vi "_sub_raw_data_analysis.vi"(11 "raw data input":u32[](array[numeric])) -> (1 "Raw-Del":u32[](array[numeric]), 2 "MAX":u32, 3 "raw data output":u32[](array[numeric]), 4 "LWA_DEL":u32, 5 "MIN":u32)   [LabVIEW 2015]
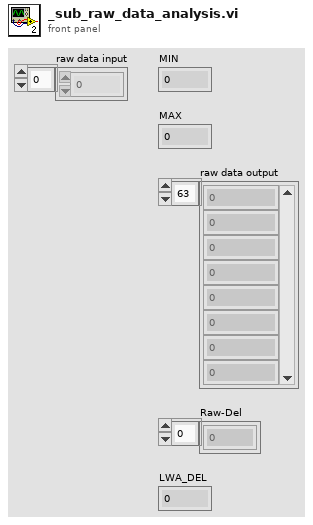
[diagram p1: front panel]
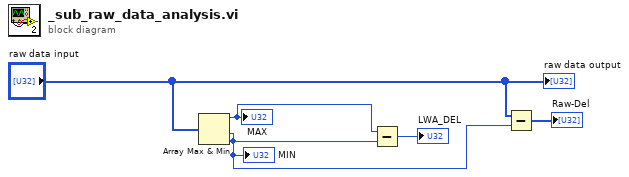
[diagram p0: block diagram]
diagram:
  n1 = Array Max & Min(array="raw data input") -> (max value=w1:u32, min value=w4:u32)  [unwired: 2 out]
  "MAX" <- w1
  "MIN" <- w4
  n2 = Subtract(x=w1, y=w4) -> (x-y=→"LWA_DEL":u32)
  n3 = Subtract(x="raw data input", y=w4) -> (x-y=→"Raw-Del":u32[])
  "raw data output" <- "raw data input"
